vi "CallHTTP.vi"(7 "Enum":enum16{"GET", "POST", "DELETE"}(ring)=enum."POST", 8 "error in (no error)":errorcluster, 9 "data":string, 10 "url":string, 11 "client handle":T1) -> (0 "error out":errorcluster, 1 "headers":string, 2 "response":string, 3 "client handle":T1)   [LabVIEW 2017]
uses:
  <vilib>/httpClient/ClientHandle.ctl
  <vilib>/httpClient/POSTBuffer.vi
  <vilib>/httpClient/LabVIEWHTTPClient.lvlib
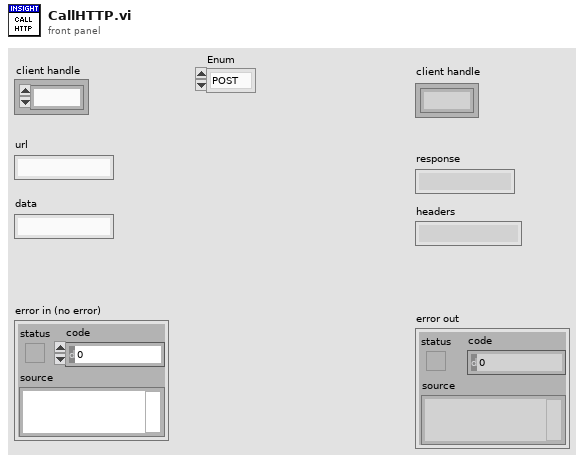
[diagram p1: front panel]
types:
  T1 = typedef "LabVIEWHTTPClient.lvlib/ClientHandle.ctl" = refnum<k1>
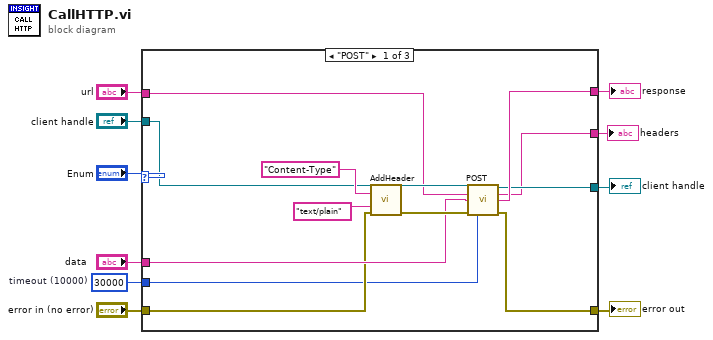
[diagram p0: block diagram]
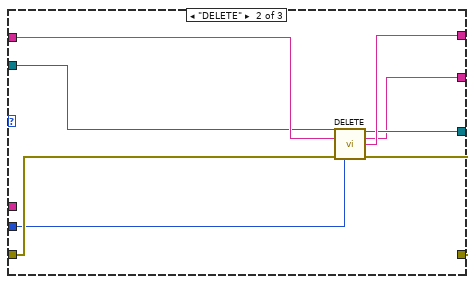
[diagram p2: hidden frame]
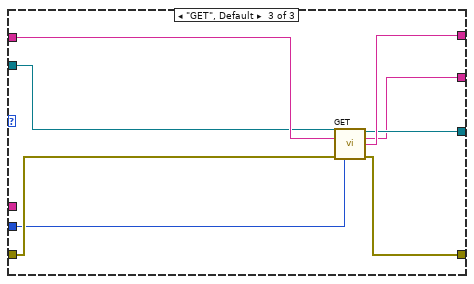
[diagram p3: hidden frame]
diagram:
  w3 = 30000  # timeout (10000)
  n1 = case shown="\"POST\"" "Enum" {
    tunnel: "url" -> [w17 w30 w38]
    tunnel: "error in (no error)" -> [w16 w27 w37]
    tunnel: [w19 w31 w39] -> w9
    tunnel: "data" -> [w18 _ _]
    tunnel: [w15 w26 w36] -> w8
    tunnel: "client handle" -> [w13 w29 w35]
    tunnel: [w14 w28 w34] -> w4
    tunnel: w3 -> [w12 w25 w33]
    tunnel: [w11 w24 w32] -> w1
    frame "POST" {
      n2 = call <vilib>:"AddHeader.vi"("client handle"=w13, "header"="Content-Type", "value"="text/plain", "error in (no error)"=w16) -> ("client handle out"=w20:T1, "error out"=w21:errorcluster)  [unwired: 10 in]
      n3 = call-poly <vilib>:"POST.vi"("client handle"=w20, "url"=w17, "buffer"=w18, "error in (no error)"=w21, "timeout (10000)"=w12) -> ("client handle out"=w14:T1, "headers"=w11:string, "body"=w19:string, "error out"=w15:errorcluster)  [unwired: 7 in]
    }
    frame "DELETE" {
      n4 = call <vilib>:"DELETE.vi"("client handle"=w29, "url"=w30, "error in (no error)"=w27, "timeout (10000)"=w25) -> ("client handle out"=w28:T1, "headers"=w24:string, "body"=w31:string, "error out"=w26:errorcluster)  [unwired: 8 in]
    }
    frame "GET", Default {
      n5 = call <vilib>:"GET.vi"("client handle"=w35, "url"=w38, "error in (no error)"=w37, "timeout (10000)"=w33) -> ("client handle out"=w34:T1, "headers"=w32:string, "body"=w39:string, "error out"=w36:errorcluster)  [unwired: 8 in]
    }
  }
  "response" <- w9
  "error out" <- w8
  "client handle" <- w4
  "headers" <- w1
